vi "CreatePizza.vi"(8 "error in (no error)":errorcluster, 10 "PizzaId":T1, 11 "PizzaStore":refnum<class "PizzaStore.lvclass">) -> (0 "error out":errorcluster, 2 "Pizza":refnum<class "Pizza.lvclass">, 3 "PizzaStore":refnum<class "PizzaStore.lvclass">)   [LabVIEW 2020, in "FactoryMethod.lvlib" / "PizzaFactoryMethod.lvlib" / "PizzaStore.lvclass"]
uses:
  PizzaStore.lvclass
  Pizza/Pizza.lvclass
  TypeDef/PizzaId.ctl
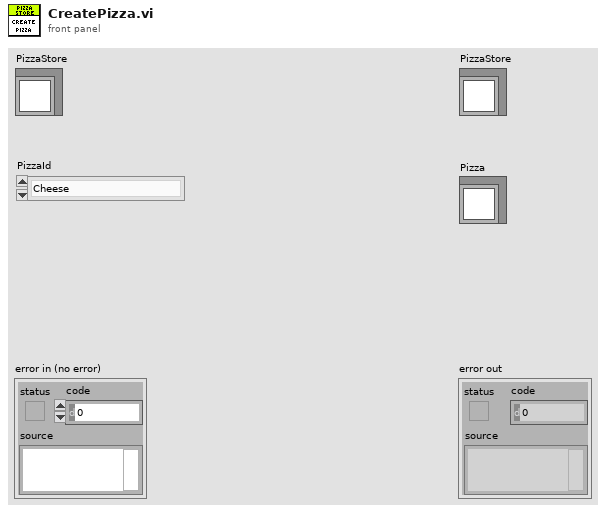
[diagram p1: front panel]
types:
  T1 = typedef "FactoryMethod.lvlib/PizzaFactoryMethod.lvlib/PizzaStore.lvclass/PizzaId.ctl" = enum16{"Cheese", "Clam", "Pepperoni", "Veggie"}
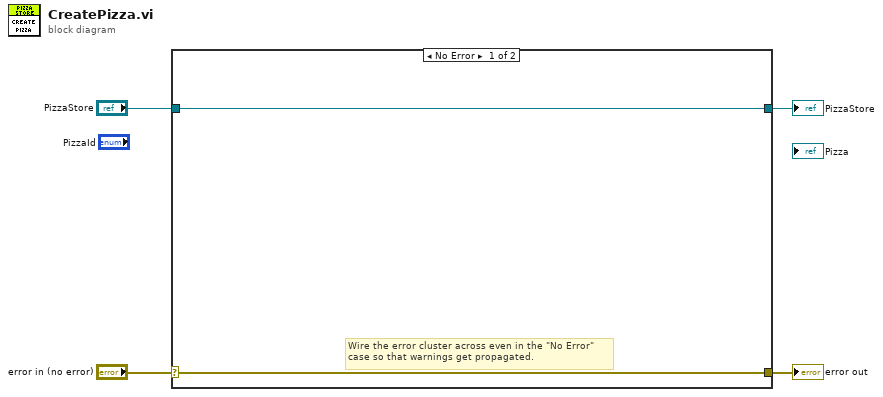
[diagram p0: block diagram]
diagram:
  n1 = case shown="No Error" "error in (no error)" {
    selector: "error in (no error)" -> [w5 w8]
    tunnel: [w5 w8] -> w3
    tunnel: [w6 w7] -> w1
    tunnel: "PizzaStore" -> [w6 w7]
    frame No Error {
      # "Wire the error cluster across even in the \"No Error\"\ncase so that warnings get propagated."
    }
    frame Error {
    }
  }
  "error out" <- w3
  "PizzaStore" <- w1
